vi "General Polynomial Fit Coefficients.vi"(0 "Y":dbl[](array[numeric]), 1 "polynomial order":i32=2, 2 "Coefficient Constraint":cluster{"order":i32, "coefficient":dbl}[](array[cluster]), 5 "X":dbl[](array[numeric]), 7 "Weight":dbl[](array[numeric]), 9 "tolerance":dbl=0.0001, 11 "method":T2 items=["Least Square", "Least Absolute Residual", "Bisquare"], 13 "algorithm":T1 items=["SVD", "Givens", "Givens2", "Householder", "LU Decomposition", "Cholesky", "SVD for Rank Deficient H"]) -> (4 "Polynomial Coefficients":dbl[](array[numeric]), 15 "error":i32)   [LabVIEW 2018, in "NI_AALPro.lvlib"]
doc: "Returns the <B>Polynomial Coefficients</B> of the general polynomial fit for a data set (<B>X</B>, <B>Y</B>) using the Least Square, Least Absolute Residue, or Bisquare methods."
uses:
  <vilib>/Analysis/NI_AALPro.lvlib
  <vilib>/Analysis/6fits.llb/Curve Fitting Criteria.ctl
  <vilib>/Analysis/6fits.llb/General Linear Fit Algorithm.ctl
panel:
  # "General Polynomial Fit Coefficients"
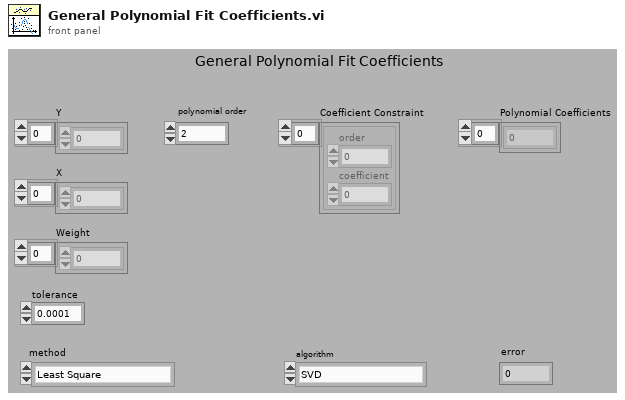
[diagram p1: front panel]
types:
  T1 = typedef "NI_AALPro.lvlib/General Linear Fit Algorithm.ctl" = u16
  T2 = typedef "NI_AALPro.lvlib/Curve Fitting Criteria.ctl" = u16
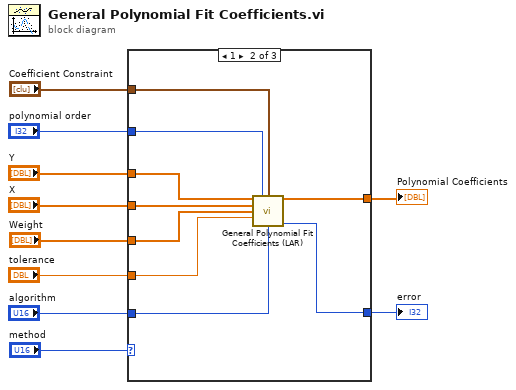
[diagram p0: block diagram]
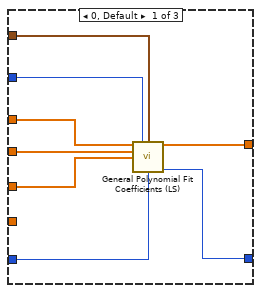
[diagram p2: hidden frame]
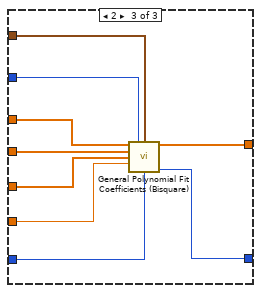
[diagram p3: hidden frame]
diagram:
  n1 = case shown="1" "method" {
    tunnel: "Coefficient Constraint" -> [w12 w20 w29]
    tunnel: "Y" -> [w18 w27 w36]
    tunnel: "X" -> [w17 w26 w35]
    tunnel: "Weight" -> [w16 w25 w34]
    tunnel: "polynomial order" -> [w11 w19 w28]
    tunnel: "algorithm" -> [w15 w23 w32]
    tunnel: [w13 w21 w30] -> w4
    tunnel: [w14 w22 w31] -> w3
    tunnel: "tolerance" -> [_ w24 w33]
    frame 0, Default {
      n2 = call "General Polynomial Fit Coefficients (LS).vi"("Y"=w18, "polynomial order"=w11, "Coefficient Constraint"=w12, "X"=w17, "Weight"=w16, "algorithm"=w15) -> ("Polynomial Coefficients"=w13:dbl[], "error"=w14:i32)  [unwired: 1 in, 7 out]
    }
    frame 1 {
      n3 = call "General Polynomial Fit Coefficients (LAR).vi"("Y"=w27, "polynomial order"=w19, "Coefficient Constraint"=w20, "X"=w26, "Weight"=w25, "tolerance"=w24, "algorithm"=w23) -> ("Polynomial Coefficients"=w21:dbl[], "error"=w22:i32)  [unwired: 1 in, 6 out]
    }
    frame 2 {
      n4 = call "General Polynomial Fit Coefficients (Bisquare).vi"("Y"=w36, "polynomial order"=w28, "Coefficient Constraint"=w29, "X"=w35, "Weight"=w34, "tolerance"=w33, "algorithm"=w32) -> ("Polynomial Coefficients"=w30:dbl[], "error"=w31:i32)  [unwired: 1 in, 6 out]
    }
  }
  "Polynomial Coefficients" <- w4
  "error" <- w3
